vi "Check temperature.vi"(8 "error in (no error)":errorcluster, 11 "Simple Device Manager in":refnum<class "Simple Device Manager.lvclass">) -> (0 "error out":errorcluster, 2 "Temperature":dbl, 3 "Simple Device Manager out":refnum<class "Simple Device Manager.lvclass">)   [LabVIEW 2020, in "Simple Device Manager.lvlib" / "Simple Device Manager.lvclass"]
uses:
  Simple Device Manager.lvclass
  Simple Device Manager.lvclass/Simple Device Manager.ctl
  Consumer Case Selector.ctl
  TALOS/TALOS_PPL.lvlibp/Ancestor/Ancestor/Infinite Message Selector.ctl
  Hardware/Simple Device/Simple Device.lvclass
  TALOS/TALOS_PPL.lvlibp
  TALOS/TALOS_PPL.lvlibp/Ancestor/Ancestor/Ancestor.lvclass
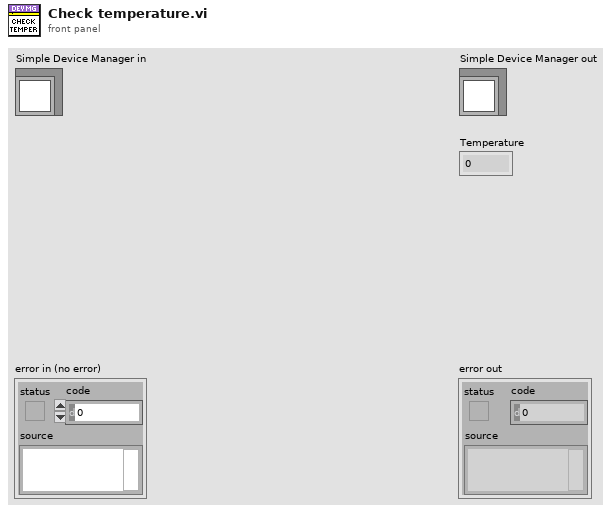
[diagram p1: front panel]
types:
  T1 = typedef "TALOS_PPL.lvlibp/Ancestor.lvlib/Ancestor.lvclass/Infinite Message Selector.ctl" = enum16{"Start", "Stop", "Check", "Flush (Stop all)", "Init"}
  T2 = typedef "Simple Device Manager.lvlib/Simple Device Manager.lvclass/Consumer Case Selector.ctl" = enum16{"Set current", "Check status", "Check temperature"}
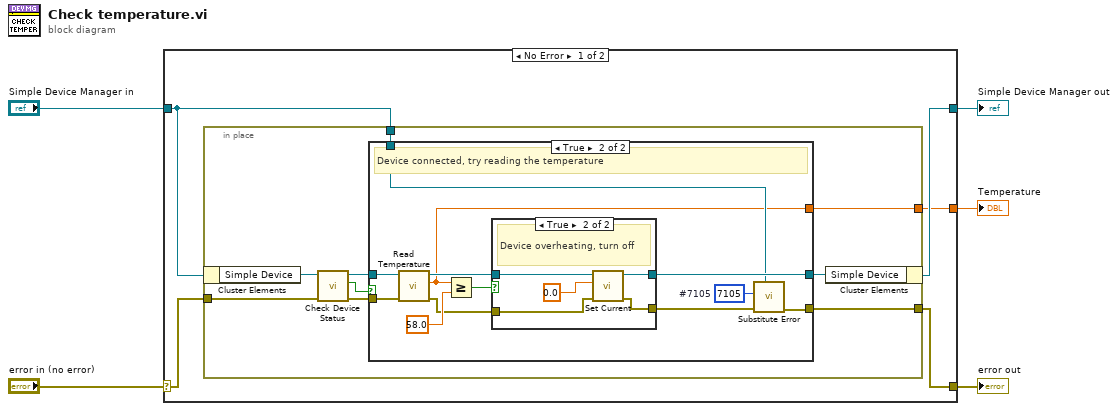
[diagram p0: block diagram]
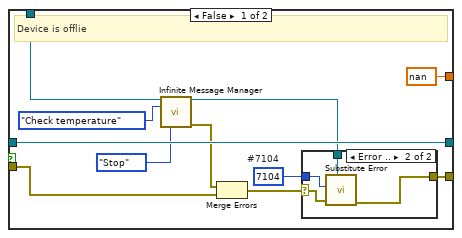
[diagram p2: hidden frame]
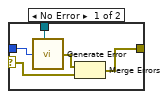
[diagram p3: hidden frame]
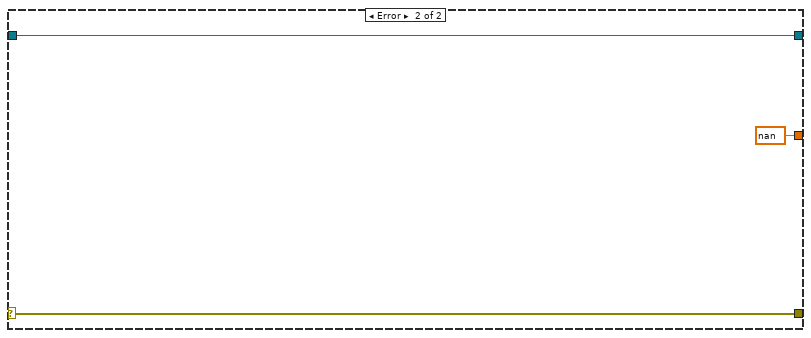
[diagram p5: hidden frame]
diagram:
  n1 = case shown="No Error" "error in (no error)" {
    selector: "error in (no error)" -> [w10 w61]
    tunnel: [w7 w61] -> w4
    tunnel: [w8 w60] -> w2
    tunnel: "Simple Device Manager in" -> [w9 w60]
    tunnel: [w6 nan ("Temperature")] -> w1
    frame No Error {
      n2 = in-place {
        in-place-border: [w18] -> w7
        in-place-border: w10 -> [w14]
        in-place-border: w9 -> [w12]
        in-place-border: [w11] -> w6
        n3 = in-place-cluster #1(w9) -> ("Simple Device"=w17:refnum<class "Simple Device.lvclass">)
        n4 = call-dynamic "Check Device Status.vi"("error in (no error)"=w14, "Simple Device in"=w17) -> ("error out"=w13:errorcluster, "Status"=w15:bool, "Simple Device out"=w16:refnum<class "Simple Device.lvclass">)  [unwired: 7 in]
        n5 = case shown="True" w15 {
          tunnel: w16 -> [w30 w51]
          tunnel: [w30 w46] -> w19
          tunnel: [w21 w43] -> w18
          tunnel: w13 -> [w25 w45]
          tunnel: w12 -> [w29 w42]
          tunnel: [nan ("Temperature") w41] -> w11
          frame False {
            w22 = 7104  # #7104
            # "Device is offlie"
            n6 = call-dynamic "Infinite Message Manager.vi"("Father of all uServices in"=w29, "Consumer Case Selector"=Consumer_Case_Selector."Check temperature", "Infinite Message Selector"=Infinite_Message_Selector."Stop") -> ("Father of all uServices out"=w20:refnum<class "Simple Device Manager.lvclass">, "error out"=w26:errorcluster)  [unwired: 10 in, 1 out]
            n7 = Merge Errors(w26, w25) -> (w23:errorcluster)
            n8 = case shown="Error .." w23 {
              selector: w23 -> [w34 w38]
              tunnel: w22 -> [w33 w39]
              tunnel: [w32 w37] -> w21
              tunnel: w20 -> [w31 w36]
              frame No Error {
                n9 = call "Generate Error.vi"("Class"=w31, "Error Code"=w33) -> ("error out"=w35:errorcluster)  [unwired: 5 in]
                n10 = Merge Errors(w35, w34) -> (w32:errorcluster)
              }
              frame Error {
                n11 = call "Substitute Error.vi"("LabVIEW Object"=w36, "error in (no error)"=w38, "Error Code"=w39) -> ("error out"=w37:errorcluster)  [unwired: 8 in]
              }
            }
          }
          frame True {
            w40 = 7105  # #7105
            # "Device connected, try reading the temperature"
            n12 = call-dynamic "Read Temperature.vi"("error in (no error)"=w45, "Simple Device in"=w51) -> ("error out"=w47:errorcluster, "Temperature"=w41:dbl, "Simple Device out"=w48:refnum<class "Simple Device.lvclass">)  [unwired: 7 in]
            n13 = Greater Or Equal?(x=w41, y=58.0) -> (x >= y?=w49:bool)
            n14 = case shown="True" w49 {
              tunnel: w48 -> [w53 w58]
              tunnel: w47 -> [w52 w56]
              tunnel: [w52 w55] -> w44
              tunnel: [w53 w54] -> w46
              frame False {
              }
              frame True {
                # "Device overheating, turn off"
                n15 = call-dynamic "Set Current.vi"("error in (no error)"=w56, "Current [mA]"=0.0, "Simple Device in"=w58) -> ("error out"=w55:errorcluster, "Simple Device out"=w54:refnum<class "Simple Device.lvclass">)  [unwired: 7 in]
              }
            }
            n16 = call "Substitute Error.vi"("LabVIEW Object"=w42, "error in (no error)"=w44, "Error Code"=w40) -> ("error out"=w43:errorcluster)  [unwired: 8 in]
          }
        }
        n17 = in-place-cluster #1("Simple Device"=w19) -> (w8:refnum<class "Simple Device Manager.lvclass">)
      }
    }
    frame Error {
    }
  }
  "error out" <- w4
  "Simple Device Manager out" <- w2
  "Temperature" <- w1
